vi "Initialize Instrument.vi"(8 "error in":errorcluster, 9 "Config Setting":variant, 10 "Initial Setting":variant, 11 "Abstract Instrument":refnum<class "Abstract Instrument.lvclass">) -> (0 "error out":errorcluster, 2 "Found?":bool, 3 "Abstract Instrument out":refnum<class "Abstract Instrument.lvclass">)   [LabVIEW 2025, in "Abstract Engine.lvlib" / "Abstract Instrument.lvclass"]
uses:
  Abstract Instrument.lvclass
  <vilib>/Utility/error.llb/DialogType.ctl
  Abstract Instrument.lvclass/Abstract Instrument.ctl
  Write error cluster.vi
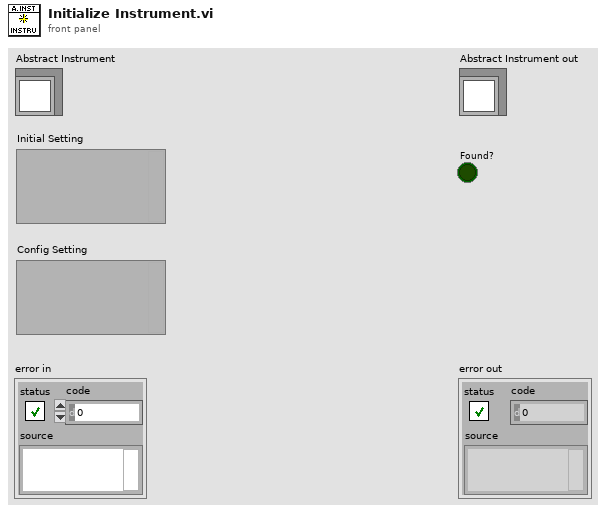
[diagram p1: front panel]
types:
  T1 = typedef "DialogType.ctl" = u16
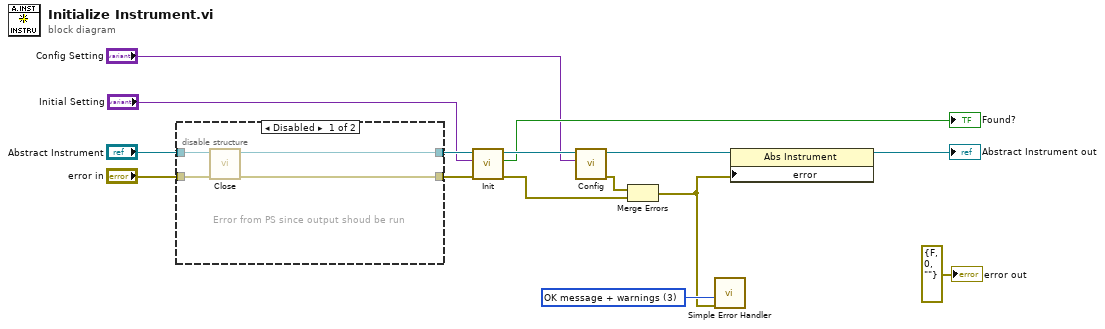
[diagram p0: block diagram]
diagram:
  w4 = T1 3 items=["no dialog", "OK message", "continue or stop message", "OK message + warnings", "continue/stop + warnings"] ("type of dialog (OK msg:1)")
  n1 = disable-structure shown="Disabled" {
    disable-tunnel: "error in" -> [w19 w20]
    disable-tunnel: "Abstract Instrument" -> [w18 w21]
    disable-tunnel: [w17 w21] -> w13
    disable-tunnel: [w16 w20] -> w12
    frame Disabled {
      # "Error from PS since output shoud be run"
      n2 = call-dynamic "Close.vi"("error in (no error)"=w19, "Abstract Instrument in"=w18) -> ("error out"=w16:errorcluster, "Abstract Instrument out"=w17:refnum<class "Abstract Instrument.lvclass">)  [unwired: 8 in]
    }
    frame Enabled {
    }
  }
  n3 = call-dynamic "Init.vi"("error in (no error)"=w12, "Initial Setting"="Initial Setting", "Abstract Instrument in"=w13) -> ("error out"=w5:errorcluster, "Found?"=→"Found?":bool, "Abstract Instrument out"=w11:refnum<class "Abstract Instrument.lvclass">)  [unwired: 6 in]
  n4 = call-dynamic "Config.vi"("Config Setting"="Config Setting", "Abstract Instrument in"=w11) -> ("error out"=w6:errorcluster, "Abstract Instrument out"=w7:refnum<class "Abstract Instrument.lvclass">)  [unwired: 8 in]
  n5 = Merge Errors(w6, w5) -> (w3:errorcluster)
  n6 = call <vilib>:"Simple Error Handler.vi"("type of dialog (OK msg:1)"=w4, "error in (no error)"=w3) -> ()  [unwired: 3 in, 5 out]
  n7 = property class="Abs Instrument"(reference=w7, "error"=w3) -> (reference out=→"Abstract Instrument out":refnum<class "Abstract Instrument.lvclass">)  [unwired: 1 in, 1 out]
  "error out" <- errorcluster {"status"=FALSE, "code"=0, "source"=""} ("error out")
